vi "FallingEdgeDetect.vi"(1 "Input":bool) -> (0 "Output":bool)   [LabVIEW 2013]
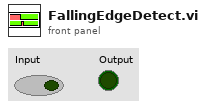
[diagram p1: front panel]
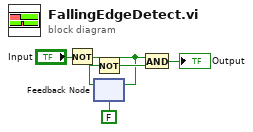
[diagram p0: block diagram]
diagram:
  n1 = Not(x="Input") -> (.not. x?=w1:bool)
  n2 = feedback #1(FALSE) -> (w4:bool)
  n3 = Not(x=w4) -> (.not. x?=w3:bool)
  n4 = feedback-in #1(w1) -> ()
  n5 = And(x=w1, y=w3) -> (x .and. y?=→"Output":bool)
